vi "userEnterCurrentSetup.vi"(7 "User input grating?":bool=TRUE, 8 "error in (no error)":errorcluster, 11 "Default wavelength (nm) 2":dbl=300.0 caption="Monochromator readout" min=261.0 max=1090.0 step=0.1 format="%#g") -> (0 "error out":errorcluster, 2 "Grating mode":T1=enum."Visible", 3 "Current wavelength (nm)":dbl=300.0)   [LabVIEW 2017]
doc: "Displays a standard dialog box that prompts users to enter information, such as a user name and password.\n--------------------\n\nThis Express VI is configured as follows:\n\nMessage to Display to the User:Please enter the number from the monochromator. \nThe inputs are: \nNumber: Monochromator readout"
uses:
  Controls/Grating.ctl
  Monochromator.lvlib
panel:
  in  "Grating":T1
  in  "Wavelength (nm)":dbl=300.0 caption="Monochromator readout" min=261.0 max=1090.0 step=0.1 format="%#g"
  in  "Enable":bool=TRUE
  in  "Cancel":bool
  out "OK":bool=TRUE
  in  "OK":bool caption="OK1"
  # "Please enter the current \nmonochromator settings:"
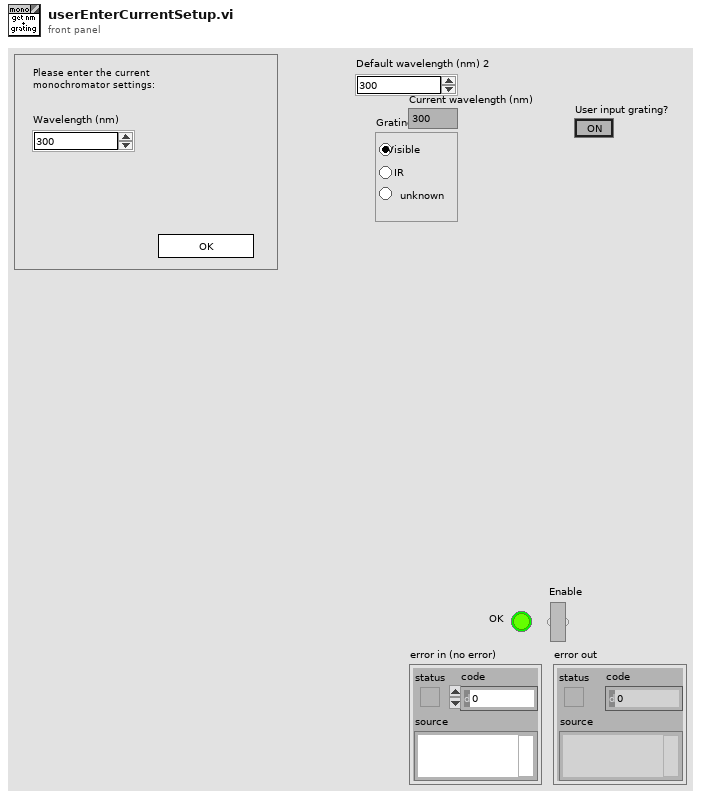
[diagram p1: front panel]
types:
  T1 = typedef "Monochromator.lvlib/Grating.ctl" = enum32{"unknown", "Visible", "IR"}
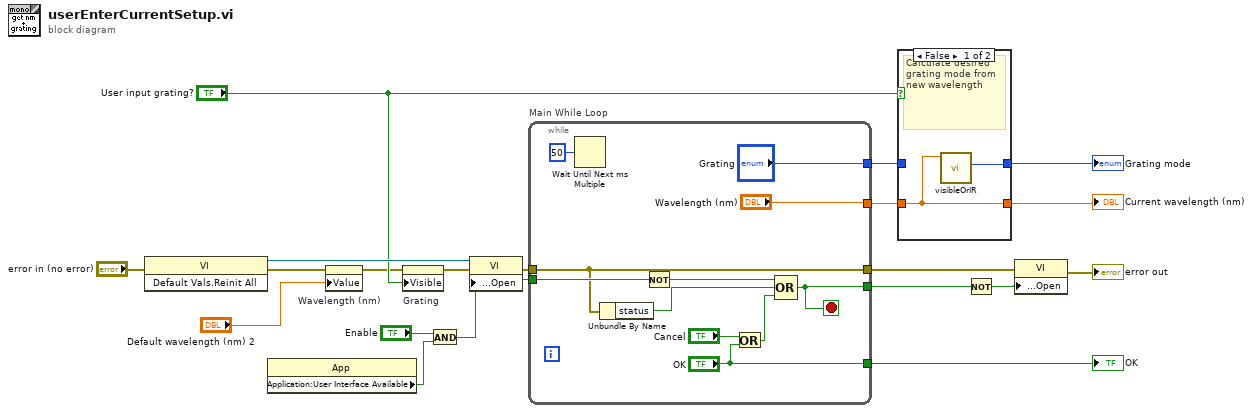
[diagram p0: block diagram]
diagram:
  n1 = invoke class="VI" method="Default Vals.Reinit All"(error in="error in (no error)") -> (reference out=w11:refnum<vi>, error out=w3:errorcluster)  [unwired: 2 in, 1 out]
  n2 = property class="App"() -> ("Application:User Interface Available"=w12:bool)  [unwired: 2 in, 2 out]
  n3 = property on="Wavelength (nm)" class="DigNum (strict)"(error in=w3, "Value"="Default wavelength (nm) 2") -> (error out=w2:errorcluster)  [unwired: 1 in, 1 out]
  n4 = property on="Grating" class="RadioBtnsControl (strict)"(error in=w2, "Visible"="User input grating?") -> (error out=w8:errorcluster)  [unwired: 1 in, 1 out]
  n5 = And(x="Enable", y=w12) -> (x .and. y?=w13:bool)
  n6 = property class="VI"(reference=w11, error in=w8, "Front Panel Window:Open"=w13) -> (error out=w17:errorcluster)  [unwired: 1 out]
  n7 = while "Main While Loop" {
    tunnel: ["OK"] -> w20
    tunnel: w13 -> [w29]
    tunnel: [w27] -> w18
    tunnel: w17 -> [w26]
    tunnel: [w26] -> w16
    tunnel: ["Wavelength (nm)"] -> w7
    tunnel: ["Grating"] -> w5
    stop <- w27 stop-if-true
    n8 = Wait Until Next ms Multiple(millisecond multiple=u32 50) -> ()  [unwired: 1 out]
    n9 = Unbundle By Name(w26) -> ("status"=w24:bool)
    n10 = Not(x=w29) -> (.not. x?=w28:bool)
    n11 = Or(x="Cancel", y="OK") -> (x .or. y?=w25:bool)
    n12 = Compound Arithmetic op=OR(w28, w24, w25) -> (w27:bool)
  }
  "OK" <- w20
  n13 = case shown="False" "User input grating?" {
    tunnel: w7 -> [w33 w34]
    tunnel: [w33 w34] -> w4
    tunnel: [w32 w35] -> w9
    tunnel: w5 -> [_ w35]
    frame False {
      # "Calculate desired grating mode from new wavelength"
      n14 = call "visibleOrIR.vi"("Wavelength (nm)"=w33) -> ("IR/visible"=w32:T1)  [unwired: 9 in, 1 out]
    }
    frame True {
      # "User inputs current grating mode (for initialisation)"
    }
  }
  "Grating mode" <- w9
  "Current wavelength (nm)" <- w4
  n15 = Not(x=w18) -> (.not. x?=w19:bool)
  n16 = property class="VI"(error in=w16, "Front Panel Window:Open"=w19) -> (error out=→"error out":errorcluster)  [unwired: 1 in, 1 out]
